vi "Lookup Target Channels.vi"(6 "VolatusAPI":refnum<class "VolatusAPI.lvclass">, 8 "error in (no error)":errorcluster, 11 "LoggingControl in":refnum<class "LoggingControl.lvclass">) -> (0 "error out":errorcluster, 3 "LoggingControl out":refnum<class "LoggingControl.lvclass">)   [LabVIEW 2020, in "VolatusGUIElements.lvlib" / "LoggingControl.lvclass"]
uses:
  LoggingControl.lvclass
  Volatus/VolatusAPI/VolatusAPI.lvclass
  LoggingControl.lvclass/LoggingControl.ctl
  Volatus/VolatusAPI/VolatusAPI.lvclass/VolatusAPI.ctl
  VolatusConfig/VolatusConfigElement/VolatusConfigElement.lvclass/VolatusConfigElement.ctl
  lv-vecto/Vecto/Channel STR/Channel STR.lvclass/Channel STR.ctl
  VolatusConfig/VolatusConfigElement/Element.vi
  lv-vecto/Vecto/Channel STR/Init.vi
  VolatusConfig/Node/Node Config.lvclass
  C:/dev/lv20CE/relink/lv-volatus/VolatusConfig/VolatusConfigElement/VolatusConfigElement.lvclass
  lv-cdm/CDM-Config/Config Element/Owner.vi
  lv-cdm/CDM-Config/Config Manager/Lookup Descendant.vi
  lv-vecto/Vecto/Channel STR/Channel STR.lvclass
  VolatusConfig/Cluster/Cluster Config.lvclass
  VolatusConfig/VolatusConfigElement/VolatusConfigElement.lvclass
  lv-cdm/CDM-Config/Config Filter/Config Lookup.lvclass
  VolatusConfig/Channel/Channel Config.lvclass
  lv-vecto/Vecto/Group DBL/Group DBL.lvclass
  C:/dev/lv20CE/relink/lv-volatus/VolatusConfig/Node/Node Config.lvclass
  C:/dev/lv20CE/relink/lv-vecto/Vecto/Group/Group.lvclass
  C:/dev/lv20CE/relink/lv-vecto/Vecto/Group DBL/Group DBL.lvclass
  lv-vecto/Vecto/Channel DBL/Channel DBL.lvclass
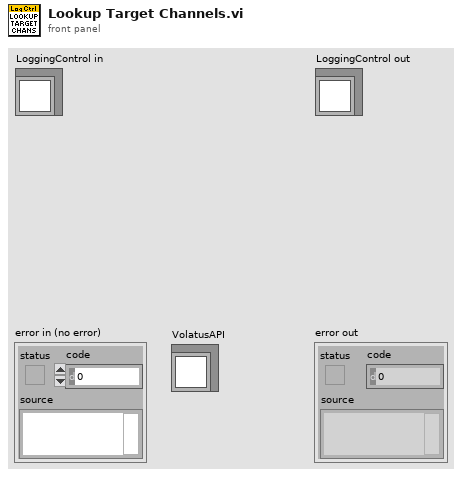
[diagram p1: front panel]
types:
  T1 = typedef "VectoConfig.lvlib/Channel Info.ctl" = cluster{"Name":string, "Group":string, "Owning Node":string, "Owning Task":string, "Resource":string}
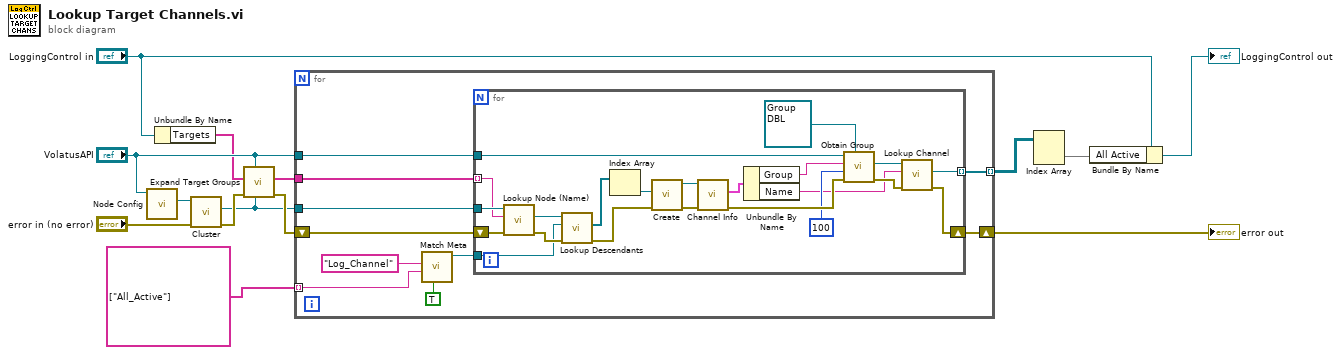
[diagram p0: block diagram]
diagram:
  n1 = call "Node Config.vi"("VolatusAPI in"="VolatusAPI") -> ("Node Config"=w12:refnum<class "Node Config.lvclass">)  [unwired: 9 in, 1 out]
  n2 = Unbundle By Name("LoggingControl in") -> ("Targets"=w4:string[])
  n3 = call "Cluster.vi"("error in (no error)"="error in (no error)", "Node in"=w12) -> ("error out"=w2:errorcluster, "Cluster"=w1:refnum<class "Cluster Config.lvclass">)  [unwired: 7 in, 1 out]
  n4 = call "Expand Target Groups.vi"("Cluster"=w1, "VolatusAPI"="VolatusAPI", "error in (no error)"=w2, "Target Names"=w4) -> ("error out"=w14:errorcluster, "Nodes"=w3:string[])  [unwired: 6 in]
  n5 = for {
    tunnel: w1 -> [w24]
    tunnel: w3 -> [w23]
    tunnel: "VolatusAPI" -> [w21]
    tunnel: [w20] -> w7 mode=indexing
    shift-right: [w19] -> w10
    shift-left: w14 -> [w22]
    tunnel: string[] ["All_Active"] -> [w16] mode=indexing
    n6 = call "Match Meta.vi"("Exact Value (F)"=TRUE, "Value (Any)"=w16, "Name"="Log_Channel") -> ("Config Lookup out"=w17:refnum<class "Config Lookup.lvclass">)  [unwired: 7 in, 1 out]
    n7 = for {
      tunnel: w24 -> [w43]
      tunnel: w23 -> [w42] mode=indexing
      tunnel: w17 -> [w40]
      shift-right: [w26] -> w19
      shift-left: w22 -> [w39]
      tunnel: w21 -> [w33]
      tunnel: [w25] -> w20 mode=indexing
      n8 = call "Lookup Node (Name).vi"("error in (no error)"=w39, "Node Name"=w42, "Cluster in"=w43) -> ("error out"=w44:errorcluster, "Node"=w41:refnum<class "Node Config.lvclass">)  [unwired: 6 in, 1 out]
      n9 = call "Lookup Descendants.vi"("error in (no error)"=w44, "Lookup"=w40, "VolatusConfigElement in"=w41) -> ("error out"=w36:errorcluster, "Descendants"=w38:refnum<class "Config Element.lvclass">[])  [unwired: 6 in, 1 out]
      n10 = Index Array(array=w38) -> (element=w37:refnum<class "Config Element.lvclass">)  [unwired: 1 in]
      n11 = call "Create.vi"("error in (no error)"=w36, "Element"=w37) -> ("error out"=w34:errorcluster, "Channel out"=w35:refnum<class "Channel Config.lvclass">)  [unwired: 8 in]
      n12 = call "Channel Info.vi"("error in (no error)"=w34, "Channel in"=w35) -> ("error out"=w45:errorcluster, "Channel Info"=w32:T1)  [unwired: 7 in, 1 out]
      n13 = Unbundle By Name(w32) -> ("Group"=w30:string, "Name"=w27:string)
      n14 = call "Obtain Group.vi"("Group Type (Abstract)"=refnum<class "Group DBL.lvclass"> refnum ("Vecto.lvlib:StringGroup.lvclass"), "error in (no error)"=w45, "Timeout ms (5000)"=u32 100, "Group Name"=w30, "VolatusAPI in"=w33) -> ("error out"=w46:errorcluster, "Group"=w28:refnum<class "Group DBL.lvclass">)  [unwired: 4 in, 1 out]
      n15 = call "Lookup Channel.vi"("error in (no error)"=w46, "Channel Name"=w27, "Group in"=w28) -> ("error out"=w26:errorcluster, "Channel"=w25:refnum<class "Channel DBL.lvclass">)  [unwired: 6 in, 1 out]
    }
  }
  "error out" <- w10
  n16 = Index Array(array=w7) -> (element=w6:refnum<class "Channel DBL.lvclass">[])  [unwired: 2 in]
  n17 = Bundle By Name(cluster="LoggingControl in", "All Active"=w6) -> (→"LoggingControl out":refnum<class "LoggingControl.lvclass">)
